vi "S4ICS Batch Command no delay.vi"() -> ()   [LabVIEW 2018]
panel:
  out "cmd #":i32
  out "current time":timestamp format="%<%H:%M:%S%3u\n%Y/%m/%d>T"
  out "batch cmd":string
  in  "batch file":string="WPROT" caption="Batch File Name"
  in  "allin":T1={"s4icsIP"="localhost", "s4icsPort"=54165, "mech name"="", "cmd"=[], "log"=refnum} {"s4icsPort" min=1025 step=1}
  in  "stop":bool
  # "S4ICS Batch Command"
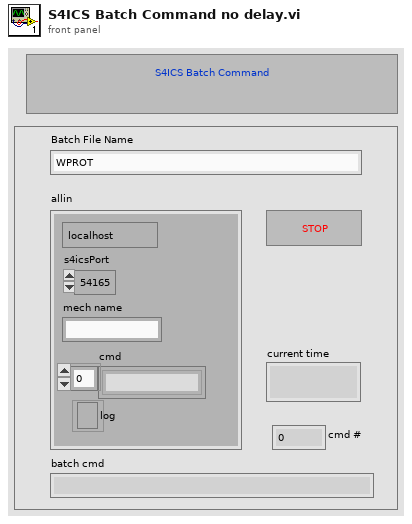
[diagram p1: front panel]
types:
  T1 = cluster{"s4icsIP":string, "s4icsPort":u16, "mech name":string, "cmd":string[], "log":refnum<file>}
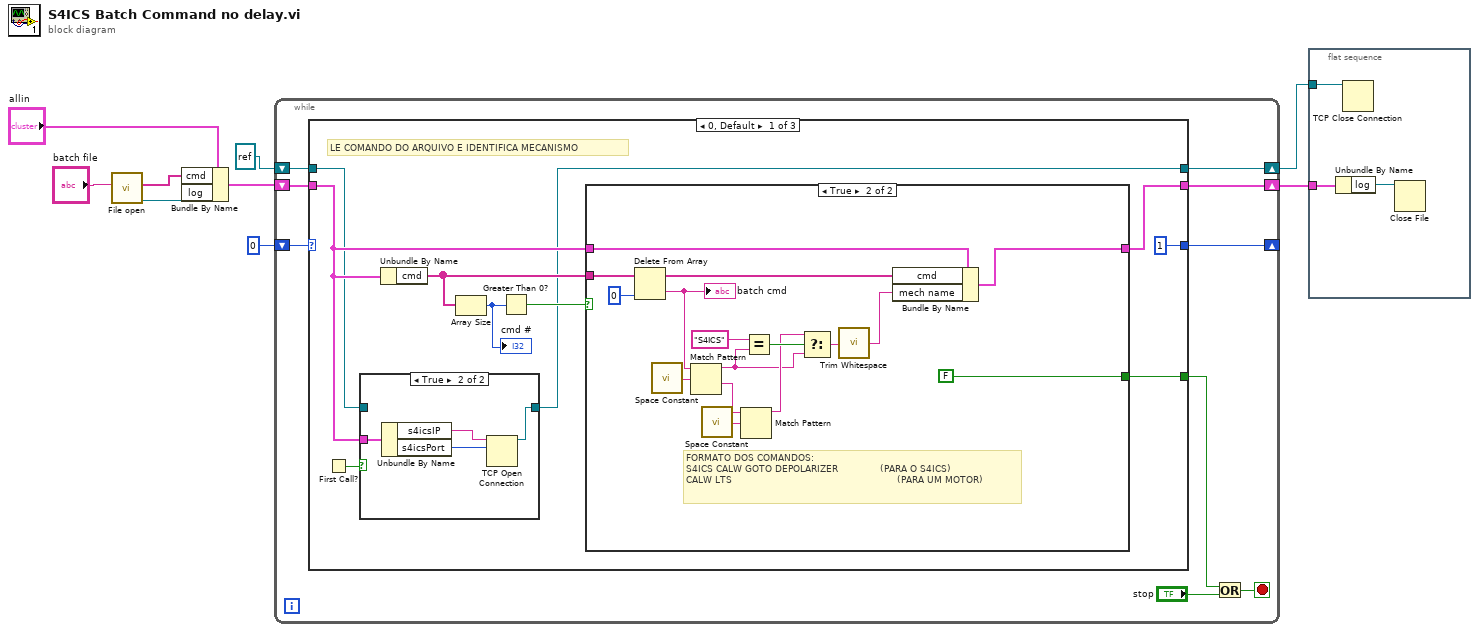
[diagram p0: block diagram]
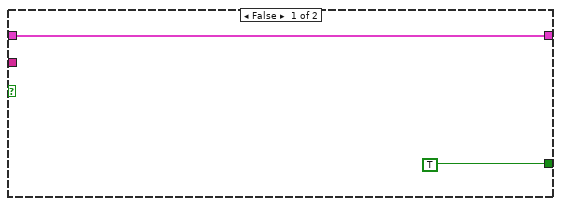
[diagram p3: hidden frame]
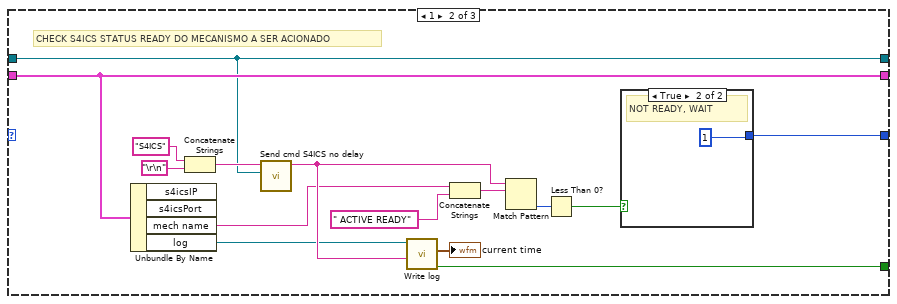
[diagram p4: hidden frame]
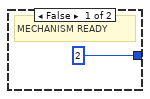
[diagram p5: hidden frame]
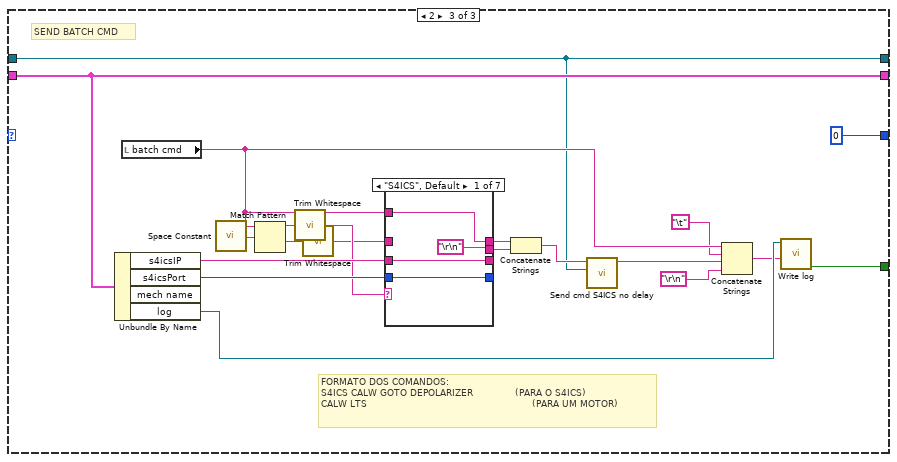
[diagram p6: hidden frame]
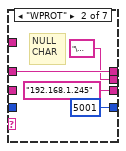
[diagram p7: hidden frame]
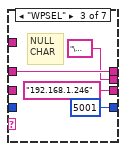
[diagram p8: hidden frame]
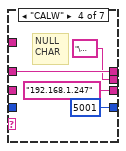
[diagram p9: hidden frame]
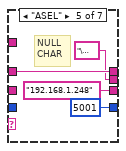
[diagram p10: hidden frame]
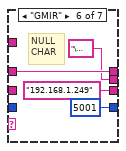
[diagram p11: hidden frame]
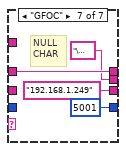
[diagram p12: hidden frame]
diagram:
  n1 = call "File open.vi"("file name"="batch file") -> ("log"=w7:refnum<file>, "cmd"=w6:string[])  [unwired: 9 in]
  n2 = Bundle By Name(cluster="allin", "cmd"=w6, "log"=w7) -> (w8:T1)
  n3 = while {
    shift-right: [w17] -> _
    shift-left: u8 0 -> [w18]
    shift-right: [w15] -> w4
    shift-left: w8 -> [w16]
    shift-right: [w10] -> w1
    shift-left: refnum<k5> refnum ("connection ID") -> [w11]
    stop <- w13 stop-if-true
    n4 = case shown="0, Default" w18 {
      tunnel: [u8 1 ("x+1") w53 u8 0 ("x+1")] -> w17
      tunnel: w16 -> [w22 w61 w86]
      tunnel: [w24 w61 w86] -> w15
      tunnel: [w26 w59 w79] -> w12
      tunnel: w11 -> [w19 w52 w69]
      tunnel: [w20 w52 w69] -> w10
      frame 0, Default {
        # "LE COMANDO DO ARQUIVO E IDENTIFICA MECANISMO"
        n5 = First Call?() -> (First Call?: T/F=w21:bool)
        n6 = case shown="True" w21 {
          tunnel: w22 -> [_ w31]
          tunnel: [w29 w30] -> w20
          tunnel: w19 -> [w29 _]
          frame False {
          }
          frame True {
            n7 = Unbundle By Name(w31) -> ("s4icsIP"=w32:string, "s4icsPort"=w33:u16)
            n8 = TCP Open Connection(address=w32, remote port or service name=w33) -> (connection ID=w30:refnum<k5>)  [unwired: 1 in, 3 out]
          }
        }
        n9 = Unbundle By Name(w22) -> ("cmd"=w23:string[])
        n10 = Array Size(array=w23) -> (size(s)=w28:i32)
        "cmd #" <- w28
        n11 = Greater Than 0?(x=w28) -> (x > 0?=w27:bool)
        n12 = case shown="True" w27 {
          tunnel: w23 -> [_ w51]
          tunnel: w22 -> [w35 w50]
          tunnel: [w35 w49] -> w24
          tunnel: [TRUE FALSE] -> w26
          frame False {
          }
          frame True {
            # "FORMATO DOS COMANDOS:\nS4ICS CALW GOTO DEPOLARIZER              (PARA O S4ICS)\nCALW LTS                                                       (PARA UM MOTOR)"
            n13 = Delete From Array(array=w51, index=0) -> (deleted portion=w45:string, array with subset deleted=w48:string[])  [unwired: 1 in]
            "batch cmd" <- w45
            n14 = call <vilib>:"Space Constant.vi"() -> ("String"=w46:string)
            n15 = Match Pattern(string=w45, regular expression=w46) -> (before substring=w38:string, after substring=w42:string)  [unwired: 1 in, 2 out]
            n16 = call <vilib>:"Space Constant.vi"() -> ("String"=w43:string)
            n17 = Match Pattern(string=w42, regular expression=w43) -> (before substring=w39:string)  [unwired: 1 in, 3 out]
            n18 = Equal?(x="S4ICS", y=w38) -> (x = y?=w40:bool)
            n19 = Select(t=w39, s=w40, f=w38) -> (s? t:f=w37:string)
            n20 = call <vilib>:"Trim Whitespace.vi"("string"=w37) -> ("trimmed string"=w36:string)  [unwired: 1 in]
            n21 = Bundle By Name(cluster=w50, "cmd"=w48, "mech name"=w36) -> (w49:T1)
          }
        }
      }
      frame 1 {
        # "CHECK S4ICS STATUS READY DO MECANISMO A SER ACIONADO"
        n22 = Unbundle By Name(w61) -> ("mech name"=w56:string, "log"=w58:refnum<file>)  [unwired: 2 out]
        n23 = Concatenate Strings("S4ICS", "\r\n") -> (w64:string)
        n24 = call "Send cmd S4ICS no delay.vi"("connection ID"=w52, "data in"=w64) -> ("data out"=w60:string)  [unwired: 8 in, 1 out]
        n25 = call "Write log.vi"("text"=w60, "log file"=w58) -> ("status"=w59:bool, "current time"=→"current time":timestamp)  [unwired: 8 in]
        n26 = Concatenate Strings(w56, " ACTIVE READY") -> (w57:string)
        n27 = Match Pattern(string=w60, regular expression=w57) -> (offset past match=w63:i32)  [unwired: 1 in, 3 out]
        n28 = Less Than 0?(x=w63) -> (x < 0?=w54:bool)
        n29 = case shown="True" w54 {
          tunnel: [u8 2 ("f") u8 1 ("f")] -> w53
          frame False {
            # "MECHANISM READY"
          }
          frame True {
            # "NOT READY, WAIT"
          }
        }
      }
      frame 2 {
        # "FORMATO DOS COMANDOS:\nS4ICS CALW GOTO DEPOLARIZER              (PARA O S4ICS)\nCALW LTS                                                       (PARA UM MOTOR)"
        # "SEND BATCH CMD"
        n30 = Unbundle By Name(w86) -> ("s4icsIP"=w88:string, "s4icsPort"=w87:u16, "log"=w78:refnum<file>)  [unwired: 1 out]
        n31 = local read "batch cmd"() -> (w77:string)
        n32 = call <vilib>:"Space Constant.vi"() -> ("String"=w83:string)
        n33 = Match Pattern(string=w77, regular expression=w83) -> (before substring=w73:string, after substring=w82:string)  [unwired: 1 in, 2 out]
        n34 = call <vilib>:"Trim Whitespace.vi"("string"=w73) -> ("trimmed string"=w72:string)  [unwired: 1 in]
        n35 = call <vilib>:"Trim Whitespace.vi"("string"=w82) -> ("trimmed string"=w71:string)  [unwired: 1 in]
        n36 = case shown="\"S4ICS\", Default" w72 {
          tunnel: w88 -> [w92 _ _ _ _ _ _]
          tunnel: w87 -> [w91 _ _ _ _ _ _]
          tunnel: [w92 "192.168.1.245" ("s4icsIP") "192.168.1.246" ("s4icsIP") "192.168.1.247" ("s4icsIP") "192.168.1.248" ("s4icsIP") "192.168.1.249" ("s4icsIP") "192.168.1.249" ("s4icsIP")] -> _
          tunnel: [w91 u16 5001 ("s4icsPort") u16 5001 ("s4icsPort") u16 5001 ("s4icsPort") u16 5001 ("s4icsPort") u16 5001 ("s4icsPort") u16 5001 ("s4icsPort")] -> _
          tunnel: w71 -> [_ w94 w98 w102 w106 w110 w114]
          tunnel: w77 -> [w90 _ _ _ _ _ _]
          tunnel: [w90 w94 w98 w102 w106 w110 w114] -> w81
          tunnel: ["\r\n" "\u0000" ("search string") "\u0000" ("search string") "\u0000" ("search string") "\u0000" ("search string") "\u0000" ("search string") "\u0000" ("search string")] -> w80
          frame "S4ICS", Default {
          }
          frame "WPROT" {
            # "NULL\nCHAR"
          }
          frame "WPSEL" {
            # "NULL\nCHAR"
          }
          frame "CALW" {
            # "NULL\nCHAR"
          }
          frame "ASEL" {
            # "NULL\nCHAR"
          }
          frame "GMIR" {
            # "NULL\nCHAR"
          }
          frame "GFOC" {
            # "NULL\nCHAR"
          }
        }
        n37 = Concatenate Strings(w81, w80) -> (w84:string)
        n38 = call "Send cmd S4ICS no delay.vi"("connection ID"=w69, "data in"=w84) -> ("data out"=w76:string)  [unwired: 8 in, 1 out]
        n39 = Concatenate Strings(w77, "\t", w76, "\r\n") -> (w75:string)
        n40 = call "Write log.vi"("text"=w75, "log file"=w78) -> ("status"=w79:bool)  [unwired: 8 in, 1 out]
      }
    }
    n41 = Or(x=w12, y="stop") -> (x .or. y?=w13:bool)
  }
  n42 = flat-sequence {
    tunnel: w4 -> [w119]
    tunnel: w1 -> [w117]
    frame #0 {
      n43 = Unbundle By Name(w119) -> ("log"=w118:refnum<file>)
      n44 = TCP Close Connection(connection ID=w117) -> ()  [unwired: 2 in, 2 out]
      n45 = Close File(refnum=w118) -> ()  [unwired: 1 in, 2 out]
    }
  }
